vi "Create.vi"(8 "error in (no error)":errorcluster, 10 "Async Plugins":refnum<class "Plugin.lvclass">[](array[class]), 11 "Dispatcher type":refnum<class "Async Dispatcher.lvclass">) -> (0 "error out":errorcluster, 3 "Dispatcher out":refnum<class "Async Dispatcher.lvclass">)   [LabVIEW 2017, in "DSF Core.lvlib" / "Async Dispatcher.lvclass"]
uses:
  Async Dispatcher.lvclass
  Plugin/Plugin.lvclass
  Async Dispatcher.lvclass/Async Dispatcher.ctl
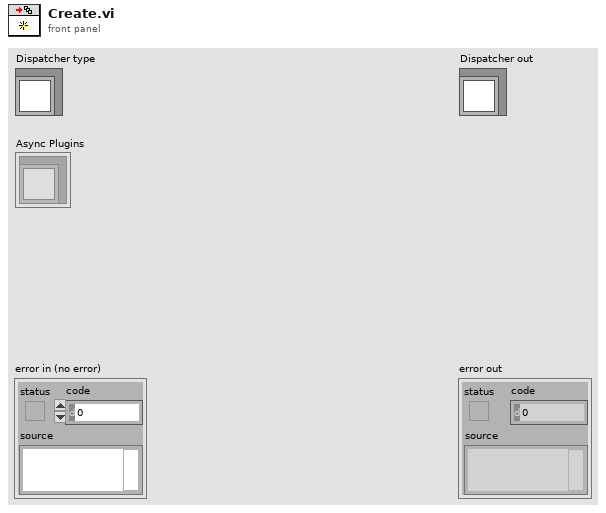
[diagram p1: front panel]
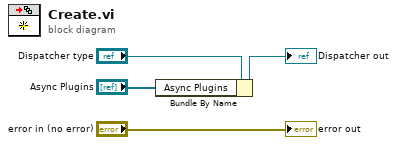
[diagram p0: block diagram]
diagram:
  n1 = Bundle By Name(cluster="Dispatcher type", "Async Plugins"="Async Plugins") -> (→"Dispatcher out":refnum<class "Async Dispatcher.lvclass">)
  "error out" <- "error in (no error)"
